vi "Dashboard Main.vi"() -> ()   [LabVIEW 2013]
uses:
  Vision/HSLRange.ctl
  <vilib>/event_ctls.llb/eventvkey.ctl
  <vilib>/Rock Robotics/WPI/Dashboard/WPI_DashboardLogging Global.vi
  <vilib>/Utility/config.llb/Write Key (String).vi
  <vilib>/Utility/config.llb/Write Key (I32).vi
  <vilib>/Utility/config.llb/NI_LVConfig.lvlib
panel:
  out "RobotIP":string
  out "Image Message":string="Timeout in Camera Communications"
  in  "Rec Mode":enum32{"Stop", "Record", "Playback"}(radio)
  in  "Dashboard Tab":T1(tab)
  in  "Camera Settings":T2={"Frame Rate"=30, "Compression"=30, "Size"=1} {"Frame Rate" scale=1.0..30.0; "Size" items=["640x480", "320x240", "160x120"]}
  out "MotorSliders R":cluster{"MotorSlide1":dbl, "MotorSlide2":dbl} {"MotorSlide2" scale=-1.0..1.0 scale format="%#_2e"; "MotorSlide1" scale=-1.0..1.0 scale format="%#_2e"}
  out "MotorChart R":cluster{"Numeric":dbl, "Numeric":dbl}(graph)
  out "MotorSliders L":T3 {"MotorSlide4 2" scale=0.0..14.0 scale format="%#_2e"; "MotorSlide2" scale=-1.0..1.0 scale format="%#_2e"; "MotorSlide1" scale=-1.0..1.0 scale format="%#_2e"}
  out "MotorChart L":T4(graph)
  out "JS1 Z":dbl(slide) scale=-1.0..1.0 scale format="%#_2e"
  out "Joystick 1":cluster{"X":dbl, "Y":dbl}[](graph)
  out "JS Buttons 1":T5
  out "JS2 Z":dbl(slide) scale=-1.0..1.0 scale format="%#_2e"
  out "Joystick 2":cluster{"X":dbl, "Y":dbl}[](graph)
  out "JS Buttons 2":T5
  out "Mode":T6(ring)=enum."Auto Disabled"
  out "Camera IP":string
  in  "DB Camera Config":bool
  out "fps":dbl format="%#.1g"
  out "Mbps":dbl format="%#.1g"
  out "Mbps 2":bool
  out "LED 1":bool
  in  "Score Limit":dbl
  in  "Minimum Area":dbl
  in  "HSL Range":T7={"Hue"={0.0, 130.10204081632654}, "Saturation"={111.88775510204081, 255.0}, "Luminance"={205.5612244897959, 255.0}} {"Luminance" scale=0.0..255.0; "Saturation" scale=0.0..255.0; "Hue" scale=0.0..255.0}
  in  "Checkbox 2":bool
  in  "Checkbox 1":bool
  in  "Test Slider":dbl(slide) scale=0.0..100.0 scale format="%#_3g"
  in  "On/Off":bool caption="Solenoid"
  in  "Test Name":u16(ring) items=["Select the test to run...", "Example Test", "-------------------------------", "List of tests is built in robot code.", "Replace with your own automated tests."]
  in  "Test Tree":string(tree)
  in  "Motor":cluster{"Value":dbl, "Enable":bool} {"Value" scale=-1.0..1.0 scale format="%#_3g"}
  out "Progress":T8 {"Test Progress" scale=0.0..100.0}
  in  "Rev/Fwd":cluster{"Forward":bool, "Reverse":bool}
  in  "Test Ring":u16(ring) items=["Auto", "Fixed indoor", "Fixed outdoor 1", "Fixed outdoor 2", "Fixed fluorescent 1", "Fixed fluorescent 2", "Hold current"]
  in  "Listbox":i32(listbox)
  out "Tree":string(tree)
  out "Camera Image":T9(plugin-control)
  in  "Enable":bool
  # "Left"
  # "Front"
  # "Right"
  # "Battery"
  # "Customize by placing controls and indicators here and name to\nmatch Dashboard Variables on robot."
  # "This tab is a great place for autonomous settings and validation.\nCustomize by placing controls and indicators here and name to\nmatch Dashboard Variables on robot."
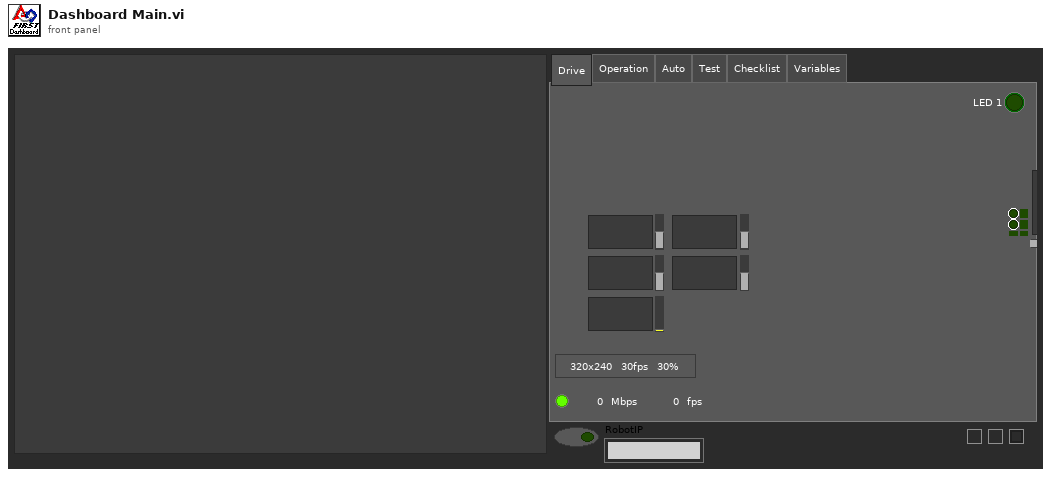
[diagram p1: front panel]
types:
  T1 = enum32{"Drive", "Operation", "Auto", "Test", "Checklist", "Variables"}
  T2 = cluster{"Frame Rate":i32, "Compression":i32, "Size":u16}
  T3 = cluster{"MotorSlide1":dbl, "MotorSlide2":dbl, "MotorSlide4 2":dbl}
  T4 = cluster{"Numeric":dbl, "Numeric":dbl, "Battery":sgl}
  T5 = cluster{bool, bool, bool, bool, bool, bool, bool, bool, bool, bool, bool, bool}
  T6 = enum8{"Tele-Op Disabled", "Tele-Op Enabled", "Auto Disabled", "Auto Enabled", "Test Disabled", "Test Enabled", ""}
  T7 = typedef "HSLRange.ctl" = cluster{"Hue":cluster{dbl, dbl}, "Saturation":cluster{dbl, dbl}, "Luminance":cluster{dbl, dbl}}
  T8 = cluster{"Test Progress":u8, "Test Progress Text":string}
  T9 = typedef "IMAQ Image.ctl" = refnum<image>
  T10 = typedef "Image Type" = u32
  T11 = typedef "Targetsss.ctl" = cluster{"Vertical Target":T12, "Horizontal Target":T12, "Valid?":bool, "Scores":T13, "Hot?":bool}
  T12 = typedef "Target Type.ctl" = cluster{"Area":dbl, "Bounding box":cluster{"BB Left":dbl, "BB Top":dbl, "BB Right":dbl, "BB Bottom":dbl}, "Center of Mass":cluster{"X Value":dbl, "Y Value":dbl}, "Equivilent Rectangle":cluster{"Width":dbl, "Height":dbl}, "Aspect Ratio":dbl, "Rectangularity":dbl, "Horizontal?":bool}
  T13 = typedef "Scores.ctl" = cluster{"Score Total":dbl, "Left Score":dbl, "Right Score":dbl, "Vertical Score":dbl, "Index":dbl}
  T14 = cluster{"BB Left":dbl, "BB Top":dbl, "BB Right":dbl, "BB Bottom":dbl}
  T15 = cluster{"Digital Inputs":bool[], "Digital Outputs":bool[]}
  T16 = cluster{"Competition mode":bool, "Robot Link":bool, "Autonomous":bool, "Enabled":bool, "E-Stop":bool, "Simulated":bool, "TestMode":bool, "Docked Window":bool}
  T17 = cluster{"Boolean Array[0]":bool, "Boolean Array[1]":bool, "Boolean Array[2]":bool, "Boolean Array[3]":bool, "Boolean Array[4]":bool, "Boolean Array[5]":bool, "Boolean Array[6]":bool, "Boolean Array[7]":bool, "Boolean Array[8]":bool, "Boolean Array[9]":bool, "Boolean Array[10]":bool, "Boolean Array[11]":bool}
  T18 = typedef "NI_LVConfig.lvlib/Config Data RefNum.ctl" = refnum<k1>
  T19 = typedef "eventvkey.ctl" = enum16{"ASCII", "Enter", "Return", "Shift", "Ctrl", "Alt", "Cmd", "Opt", "Caps", "NumLock", "Clear", "Break", "Up", "Down", "Left", "Right", "Insert", "Delete", "Home", "End", "PageUp", "PageDown", "Escape", "Help", "Pause", "ScrollLock", "F1", "F2", "F3", "F4", "F5", "F6", "F7", "F8", "F9", "F10", "F11", "F12", "F13", "F14", "F15", "F16", "F17", "F18", "F19", "F20", "F21", "F22", "F23", "F24", "Play", "VolumeUp", "VolumeDown", "Mute", "Two Byte Char"}
  T20 = cluster{"Image Size":bool, "Image Type":bool, "Pixel Value":bool, "ROI Information":bool, "Zoom Factor":bool}
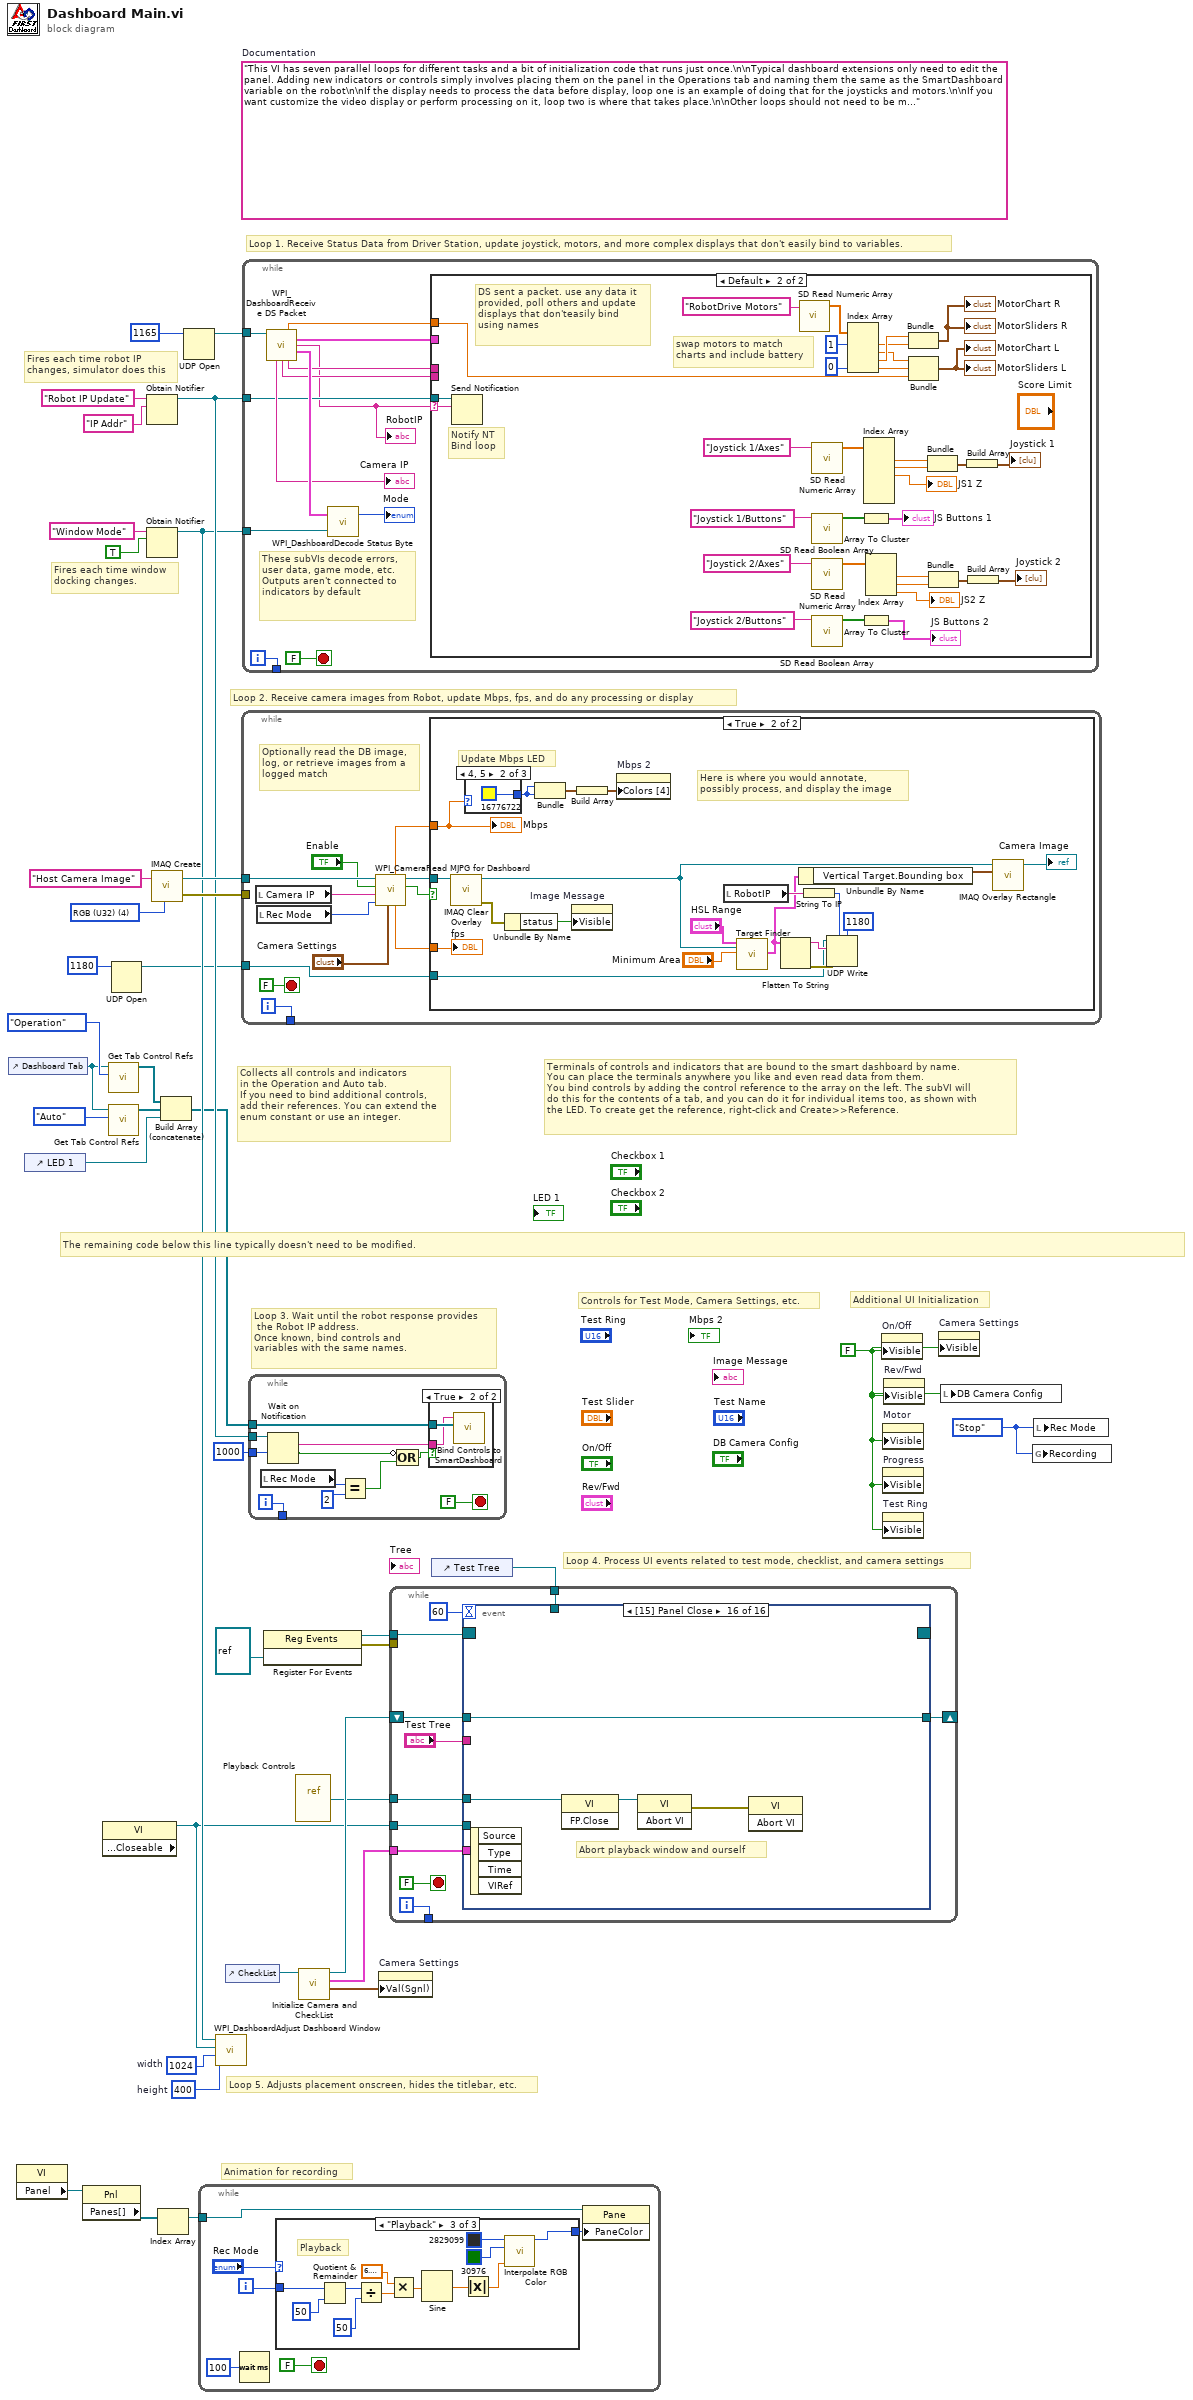
[diagram p0: block diagram]
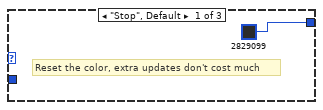
[diagram p2: hidden frame]
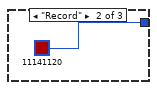
[diagram p3: hidden frame]
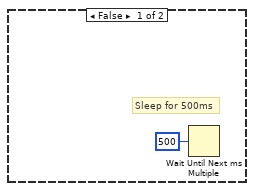
[diagram p5: hidden frame]
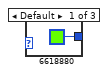
[diagram p6: hidden frame]
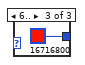
[diagram p7: hidden frame]
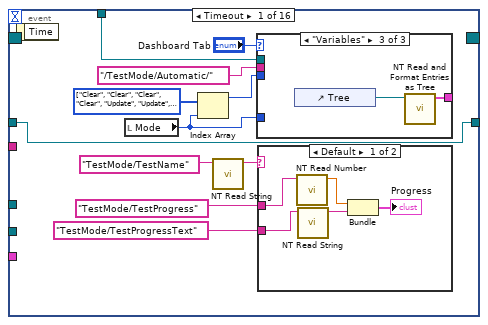
[diagram p8: hidden frame]
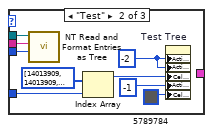
[diagram p10: hidden frame]
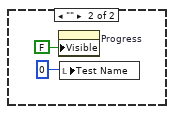
[diagram p11: hidden frame]
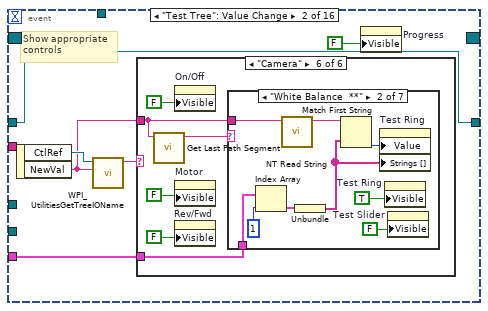
[diagram p12: hidden frame]
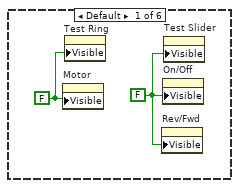
[diagram p13: hidden frame]
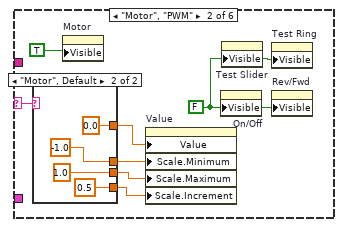
[diagram p14: hidden frame]
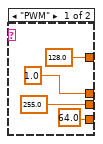
[diagram p15: hidden frame]
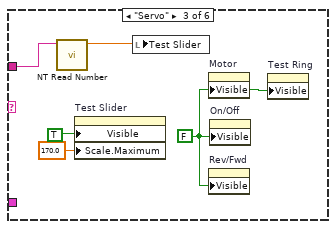
[diagram p16: hidden frame]
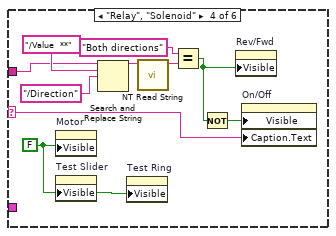
[diagram p17: hidden frame]
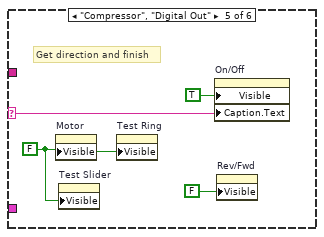
[diagram p18: hidden frame]
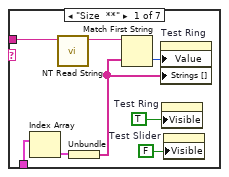
[diagram p19: hidden frame]
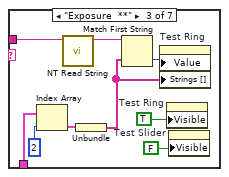
[diagram p20: hidden frame]
diagram:
  w10 = enum32{"Stop", "Record", "Playback"}."Stop" ("Rec Mode")
  w13 = 400  # height
  w14 = 1024  # width
  w27 = FALSE ("Visible")
  (unwired) "This VI has seven parallel loops for different tasks and a bit of initialization code that runs just once.\n\nTypical dashboard extensions only need to edit the panel. Adding new indicators or controls simply involves placing them on the panel in the Operations tab and naming them the same as the SmartDashboard variable on the robot\n\nIf the display needs to process the data before display, loop one is an example of doing that for the joysticks and motors.\n\nIf you want customize the video display or perform processing on it, loop two is where that takes place.\n\nOther loops should not need to be modified. They are pretty standard, and document the task they perform."  # Documentation
  w37 = T10 4 items=["Grayscale (U8)", "Grayscale (I16)", "Grayscale (SGL)", "Complex (CSG)", "RGB (U32)", "HSL (U32)", "RGB (U64)"] ("Image Type")
  # "Controls for Test Mode, Camera Settings, etc."
  # "Additional UI Initialization"
  # "Animation for recording"
  # "Fires each time robot IP\nchanges, simulator does this"
  # "Fires each time window\ndocking changes."
  # "Collects all controls and indicators\nin the Operation and Auto tab.\nIf you need to bind additional controls,\nadd their references. You can extend the\nenum constant or use an integer."
  # "The remaining code below this line typically doesn't need to be modified."
  # "Loop 4. Process UI events related to test mode, checklist, and camera settings"
  # "Terminals of controls and indicators that are bound to the smart dashboard by name.\nYou can place the terminals anywhere you like and even read data from them.\nYou bind controls by adding the control reference to the array on the left. The subVI will\ndo this for the contents of a tab, and you can do it for individual items too, as shown with\nthe LED. To create get the reference, right-click and Create>>Reference."
  # "Loop 3. Wait until the robot response provides\n the Robot IP address.\nOnce known, bind controls and\nvariables with the same names."
  # "Loop 5. Adjusts placement onscreen, hides the titlebar, etc."
  # "Loop 1. Receive Status Data from Driver Station, update joystick, motors, and more complex displays that don't easily bind to variables."
  # "Loop 2. Receive camera images from Robot, update Mbps, fps, and do any processing or display"
  n1 = control-ref of="Dashboard Tab"() -> (w8:refnum<vi>)
  n2 = property class="VI"() -> ("Panel"=w21:refnum<vi>)  [unwired: 2 in, 2 out]
  n3 = control-ref of="LED 1"() -> (w3:refnum<vi>)
  n4 = property class="Pnl"(reference=w21) -> ("Panes[]"=w22:refnum<vi>[])  [unwired: 1 in, 2 out]
  n5 = property class="VI" props=["Front Panel.Closeable"]() -> (reference out=w9:refnum<vi>)  [unwired: 2 in, 2 out]
  n6 = call <vilib>:"Get Tab Control Refs.vi"("Page Index"=T1."Operation" ("Dashboard Tab"), "TabControl in"=w8) -> ("ControlsOnPage"=w6:refnum<vi>[])  [unwired: 9 in]
  n7 = call <vilib>:"Get Tab Control Refs.vi"("Page Index"=T1."Auto" ("Dashboard Tab"), "TabControl in"=w8) -> ("ControlsOnPage"=w7:refnum<vi>[])  [unwired: 9 in]
  n8 = UDP Open(11:1180) -> (port=w2:refnum<k16>)  [unwired: 4 in, 2 out]
  n9 = Obtain Notifier(name (unnamed)="Robot IP Update", notification data type="IP Addr" ("name (unnamed)")) -> (notifier out=w31:refnum<notifier>)  [unwired: 2 in, 2 out]
  n10 = Obtain Notifier(name (unnamed)="Window Mode", notification data type=TRUE) -> (notifier out=w12:refnum<notifier>)  [unwired: 2 in, 2 out]
  n11 = call "IMAQ Create"("Image Name"="Host Camera Image", "Image Type"=w37) -> ("New Image"=w35:T9, "error out"=w34:errorcluster)  [unwired: 2 in, 1 out]
  n12 = Index Array(array=w22) -> (element=w20:refnum<vi>)  [unwired: 1 in]
  n13 = Build Array (concatenate)(w6, w7, w3) -> (w5:refnum<vi>[])
  n14 = UDP Open(11:u16 1165 ("port")) -> (port=w38:refnum<k16>)  [unwired: 2 in, 4 out]
  n15 = while {
    tunnel: w20 -> [w41]
    i -> [w44]
    stop <- FALSE stop-if-true
    n16 = Wait (ms)(milliseconds to wait=u32 100) -> ()  [unwired: 1 out]
    n17 = case shown="\"Playback\"" "Rec Mode" {
      tunnel: w44 -> [_ _ w59]
      tunnel: [u32 2829099 ("Base Color") u32 11141120 ("Target Color") w48] -> w40
      frame "Stop", Default {
        # "Reset the color, extra updates don't cost much"
      }
      frame "Record" {
      }
      frame "Playback" {
        # "Playback"
        n18 = Quotient & Remainder(x=w59, y=u32 50 ("milliseconds to wait")) -> (x-y*floor(x/y)=w55:u32)  [unwired: 1 out]
        n19 = Divide(x=w55, y=u32 50 ("milliseconds to wait")) -> (x/y=w52:dbl)
        n20 = Multiply(x=6.283185307179586, y=w52) -> (x*y=w57:dbl)
        n21 = Sine(x=w57) -> (sin(x)=w56:dbl)
        n22 = Absolute Value(x=w56) -> (abs(x)=w49:dbl)
        n23 = call "Interpolate RGB Color.vi"("Proportion"=w49, "Target Color"=u32 30976, "Base Color"=u32 2829099) -> ("Result Color"=w48:u32)  [unwired: 8 in]
      }
    }
    n24 = property class="Pane"(reference=w41, "PaneColor"=w40) -> ()  [unwired: 1 in, 2 out]
  }
  n25 = call <vilib>:"WPI_DashboardAdjust Dashboard Window.vi"("height"=w13, "width"=w14, "reference in"=w9, "Notifier in"=w12) -> ()  [unwired: 8 in]
  n26 = control-ref of="CheckList"() -> (w11:refnum<vi>)
  n27 = while {
    tunnel: w35 -> [w69]
    tunnel: w34 -> [_]
    tunnel: [w70] -> _
    tunnel: w2 -> [w60]
    i -> [w70]
    stop <- FALSE stop-if-true
    # "Optionally read the DB image,\nlog, or retrieve images from a\nlogged match"
    n28 = local read "Camera IP"() -> (w62:string)
    n29 = local read "Rec Mode"() -> (w61:enum32{"Stop", "Record", "Playback"})
    n30 = call <vilib>:"WPI_CameraRead MJPG for Dashboard.vi"("Camera Settings"="Camera Settings", "Rec Mode"=w61, "Camera IP"=w62, "Enable"="Enable", "Refnum in"=w69) -> ("Active"=w66:bool, "Refnum out"=w68:T9, "FPS"=w65:dbl, "Bandwidth (Mbps)"=w64:dbl)  [unwired: 3 in]
    n31 = case shown="True" w66 {
      tunnel: w68 -> [_ w87]
      tunnel: w64 -> [_ w86]
      tunnel: w65 -> [_ w85]
      tunnel: w60 -> [_ w81]
      frame False {
        # "Sleep for 500ms"
        n32 = Wait Until Next ms Multiple(millisecond multiple=u32 500) -> ()  [unwired: 1 out]
      }
      frame True {
        # "Here is where you would annotate,\npossibly process, and display the image"
        # "Update Mbps LED"
        n33 = call "IMAQ Clear Overlay"("Image"=w87) -> ("error out"=w91:errorcluster, "Image Out"=w77:T9)  [unwired: 2 in, 7 out]
        n34 = case shown="4, 5" w86 {
          tunnel: [u32 6618880 ("Color Box") u32 16776722 ("Color Box") u32 16716800 ("Color Box")] -> w88
          frame Default {
          }
          frame 4, 5 {
          }
          frame 6.. {
          }
        }
        n35 = Unbundle By Name(w91) -> ("status"=w92:bool)
        n36 = Bundle("Color Box"=w88, "Color Box"=w88) -> (w90:cluster{"Color Box":u32, "Color Box":u32})  [unwired: 1 out]
        n37 = property on="Image Message" class="Str"("Visible"=w92) -> ()  [unwired: 2 in, 2 out]
        n38 = Build Array(w90) -> (w89:cluster{"Color Box":u32, "Color Box":u32}[])
        n39 = property on="Mbps 2" class="Bool (strict)"("Colors [4]"=w89) -> ()  [unwired: 2 in, 2 out]
        n40 = local read "RobotIP"() -> (w78:string)
        n41 = call "Target Finder.vi"("HSL Range"="HSL Range", "Image"=w77, "Minimum Area"="Minimum Area") -> ("Targetssssss"=w74:T11)  [unwired: 16 in]
        n42 = Flatten To String(anything=w74) -> (data string=w82:string, error out=w83:errorcluster)  [unwired: 3 in, 1 out]
        n43 = Unbundle By Name(w74) -> ("Vertical Target.Bounding box"=w76:T14)
        n44 = String To IP(1:w78) -> (0:w79:u32)
        n45 = UDP Write(address=w79, port or service name=1180, connection ID=w81, data in=w82, 8:w83) -> ()  [unwired: 1 in, 2 out]
        n46 = call "IMAQ Overlay Rectangle"("Rectangle"=w76, "Image"=w77) -> ("Image Out"=→"Camera Image":T9)  [unwired: 8 in, 1 out]
        "Mbps" <- w86
        "fps" <- w85
      }
    }
  }
  n47 = while {
    tunnel: w38 -> [w106]
    tunnel: w31 -> [w101]
    tunnel: w12 -> [w105]
    tunnel: [w102] -> _
    i -> [w102]
    stop <- FALSE stop-if-true
    # "These subVIs decode errors, user data, game mode, etc.\nOutputs aren't connected to indicators by default"
    n48 = call <vilib>:"WPI_DashboardReceive DS Packet.vi"("Recv Socket"=w106) -> ("Battery"=w97:sgl, "Driver Station"=w98:T15, "Robot IP Address"=w96:string, "Status"=w107:T16, "Camera IP Address"=→"Camera IP":string, "Low Priority User Data"=w100:string, "High Priority User Data"=w99:string)  [unwired: 1 in, 7 out]
    "RobotIP" <- w96
    n49 = call <vilib>:"WPI_DashboardDecode Status Byte.vi"("Window Mode Notifier"=w105, "Status"=w107) -> ("Mode"=→"Mode":T6)  [unwired: 1 out]
    n50 = case shown="Default" w96 {
      selector: w96 -> [_ w119]
      tunnel: w101 -> [_ w120]
      tunnel: w100 -> [_ _]
      tunnel: w99 -> [_ _]
      tunnel: w98 -> [_ _]
      tunnel: w97 -> [_ w118]
      frame "0.0.0.0" {
        # "DS not sending packets, or no robot exists yet.\nDon't poll the variables"
      }
      frame Default {
        # "Notify NT\nBind loop"
        # "DS sent a packet. use any data it\nprovided, poll others and update\ndisplays that don'teasily bind\nusing names"
        # "swap motors to match\ncharts and include battery"
        n51 = Send Notification(notification=w119, notifier=w120) -> ()  [unwired: 1 in, 2 out]
        n52 = call <vilib>:"SD Read Numeric Array.vi"("Name"="RobotDrive Motors") -> ("Numeric Array"=w117:dbl[])  [unwired: 8 in, 2 out]
        n53 = call <vilib>:"SD Read Numeric Array.vi"("Name"="Joystick 1/Axes") -> ("Numeric Array"=w136:dbl[])  [unwired: 8 in, 2 out]
        n54 = call <vilib>:"SD Read Boolean Array.vi"("Name"="Joystick 1/Buttons") -> ("Boolean Array"=w138:bool[])  [unwired: 8 in, 2 out]
        n55 = call <vilib>:"SD Read Numeric Array.vi"("Name"="Joystick 2/Axes") -> ("Numeric Array"=w130:dbl[])  [unwired: 8 in, 2 out]
        n56 = call <vilib>:"SD Read Boolean Array.vi"("Name"="Joystick 2/Buttons") -> ("Boolean Array"=w129:bool[])  [unwired: 8 in, 2 out]
        n57 = Index Array(array=w117, index #1=1, index #4=0) -> (element #1=w113:dbl, element #2=w112:dbl, element #3=w114:dbl, element #4=w109:dbl)  [unwired: 2 in]
        n58 = Array To Cluster(array=w138) -> (cluster=→"JS Buttons 1":T17)
        n59 = Array To Cluster(array=w129) -> (cluster=→"JS Buttons 2":T17)
        n60 = Index Array(array=w136) -> (element #1=w133:dbl, element #2=w134:dbl, element #3=→"JS1 Z":dbl)  [unwired: 6 in, 3 out]
        n61 = Index Array(array=w130) -> (element #1=w125:dbl, element #2=w124:dbl, element #3=→"JS2 Z":dbl)  [unwired: 3 in]
        n62 = Bundle("Numeric"=w114, "Numeric"=w113) -> (→"MotorChart R" →"MotorSliders R":cluster{"Numeric":dbl, "Numeric":dbl})  [unwired: 1 in]
        n63 = Bundle("Numeric"=w112, "Numeric"=w109, "Battery"=w118) -> (→"MotorChart L" →"MotorSliders L":T4)  [unwired: 1 in]
        n64 = Bundle("Numeric"=w133, "Numeric"=w134) -> (w132:cluster{"Numeric":dbl, "Numeric":dbl})  [unwired: 1 in]
        n65 = Bundle("Numeric"=w125, "Numeric"=w124) -> (w126:cluster{"Numeric":dbl, "Numeric":dbl})  [unwired: 1 in]
        n66 = Build Array(w132) -> (→"Joystick 1":cluster{"Numeric":dbl, "Numeric":dbl}[])
        n67 = Build Array(w126) -> (→"Joystick 2":cluster{"Numeric":dbl, "Numeric":dbl}[])
      }
    }
  }
  n68 = while {
    tunnel: w5 -> [w152]
    tunnel: w31 -> [w150]
    tunnel: [w148] -> _
    tunnel: u32 1000 ("milliseconds to wait") -> [w147]
    i -> [w148]
    stop <- FALSE stop-if-true
    n69 = local read "Rec Mode"() -> (w143:enum32{"Stop", "Record", "Playback"})
    n70 = Wait on Notification(notifier=w150, timeout in ms (-1)=w147) -> (notification=w149:string, timed out?=w145:bool)  [unwired: 2 in, 2 out]
    n71 = Equal?(x=w143, y=u16 2 ("Rec Mode")) -> (x = y?=w144:bool)
    n72 = Compound Arithmetic op=OR(invert w145, w144) -> (w146:bool)
    n73 = case shown="True" w146 {
      tunnel: w152 -> [_ w154]
      tunnel: w149 -> [_ w153]
      frame False {
      }
      frame True {
        n74 = call <vilib>:"Bind Controls to SmartDashboard.vi"("Bound Control Refs"=w154, "Server IP Address"=w153) -> ()  [unwired: 10 in]
      }
    }
  }
  n75 = register-events(refnum<vi> refnum) -> (reference out=w18:refnum<event-registration>, error out=w17:errorcluster)  [unwired: 2 in]
  n76 = vi-ref "Playback Controls.vi"() -> (w19:refnum<vi>)
  n77 = call "Initialize Camera and CheckList.vi"("ListBox in"=w11) -> ("Cluster"=w25:cluster{"value":i32, "value":i32, "index":i32}, "Array"=w26:cluster{string[]}[], "File Refnum"=w24:T18)  [unwired: 8 in]
  n78 = property on="Camera Settings" class="Clust (strict)"("Val(Sgnl)"=w25) -> ()  [unwired: 2 in, 2 out]
  n79 = control-ref of="Test Tree"() -> (w23:refnum<vi>)
  n80 = while {
    tunnel: w26 -> [w162]
    shift-right: [w161] -> _
    shift-left: w24 -> [w160]
    tunnel: [w159] -> _
    tunnel: w23 -> [w158]
    tunnel: w19 -> [w157]
    tunnel: w18 -> [w156]
    tunnel: w17 -> [_]
    tunnel: w9 -> [w155]
    i -> [w159]
    stop <- FALSE stop-if-true
    n81 = event shown="[15] Panel Close" {
      selector: w156 -> [_ _ _ _ _ _ _ _ _ _ _ _ _ _ _ _]
      dyn-events: [_ _ _ _ _ _ _ _ _ _ _ _ _ w400 _ _] -> _
      timeout: u32 60 ("milliseconds to wait") -> [_ _ _ _ _ _ _ _ _ _ _ _ _ _ _ _]
      tunnel: w158 -> [w172 _ _ _ _ _ _ _ _ _ _ _ _ _ _ _]
      tunnel: "Test Tree" -> [_ _ _ _ _ _ _ _ w369 w377 w379 w383 w391 _ _ _]
      tunnel: w162 -> [_ w196 _ _ _ _ w333 w363 _ _ _ _ _ _ _ _]
      tunnel: [w166 w195 w294 w299 w307 w319 w332 w356 w368 w375 w378 w382 w390 w402 w416 w417] -> w161
      tunnel: w160 -> [w166 w195 w294 w299 w307 w319 w331 w356 w368 w375 w378 w382 w390 w402 w416 w417]
      tunnel: w157 -> [_ _ _ _ _ _ _ _ _ _ _ _ _ w403 _ w420]
      tunnel: w155 -> [_ _ _ _ _ _ _ _ _ _ _ _ _ w398 _ _]
      event Timeout {
        w171 = enum16{"Update", "Clear"}[] [enum."Clear", enum."Clear", enum."Clear", enum."Clear", enum."Update", enum."Update", enum."Clear"] items=["Update", "Clear"]
        n82 = event-data() -> ()  [unwired: 1 in, 1 out]
        n83 = local read "Mode"() -> (w169:T6)
        n84 = Index Array(array=w171, index=w169) -> (element=w170:enum16{"Update", "Clear"})
        n85 = call <vilib>:"NT Read String.vi"("Name"="TestMode/TestName") -> ("String"=w175:string)  [unwired: 9 in, 1 out]
        n86 = case shown="\"Variables\"" "Dashboard Tab" {
          tunnel: w172 -> [_ w185 _]
          tunnel: "/TestMode/Automatic/" ("Name Pattern") -> [_ w184 _]
          tunnel: w170 -> [_ w183 _]
          tunnel: w169 -> [_ w181 _]
          tunnel: [_ _ w187] -> _
          frame "Operation", Default {
          }
          frame "Test" {
            w180 = -2 ("Active Item:Row Number")
            n87 = call <vilib>:"NT Read and Format Entries as Tree.vi"("Operation"=w183, "Name Pattern"=w184, "Tree Refnum"=w185) -> ()  [unwired: 7 in, 2 out]
            n88 = Index Array(array=u32[] [14013909, 14013909, 14013909, 14013909, 14013909, 16777215, 14013909], index=w181) -> (element=w179:u32)
            n89 = property on="Test Tree" class="Tree (strict)"("Active Item Row Number"=w180, "ActiveColNum"=w180, "CellBG"=w179, "Active Item Row Number"=-1 ("Active Item:Row Number"), "CellBG"=u32 5789784 ("Color Box")) -> ()  [unwired: 2 in, 2 out]
          }
          frame "Variables" {
            n90 = control-ref of="Tree"() -> (w186:refnum<vi>)
            n91 = call <vilib>:"NT Read and Format Entries as Tree.vi"("Tree Refnum"=w186) -> ("Formatted Strings"=w187:cluster{"Name":string, "Value":string}[])  [unwired: 9 in, 1 out]
          }
        }
        n92 = case shown="Default" w175 {
          tunnel: "TestMode/TestProgress" ("Name") -> [w189 _]
          tunnel: "TestMode/TestProgressText" ("Name") -> [w188 _]
          frame Default {
            n93 = call <vilib>:"NT Read Number.vi"("Name"=w189) -> ("Numeric"=w190:dbl)  [unwired: 9 in, 1 out]
            n94 = call <vilib>:"NT Read String.vi"("Name"=w188) -> ("String"=w191:string)  [unwired: 9 in, 1 out]
            n95 = Bundle("Numeric"=w190, "String"=w191) -> (→"Progress":cluster{"Numeric":dbl, "String":string})  [unwired: 1 in]
          }
          frame "" {
            n96 = property on="Progress" class="Clust (strict)"("Visible"=FALSE) -> ()  [unwired: 2 in, 2 out]
            n97 = local write "Test Name"(u16 0) -> ()
          }
        }
      }
      event "Test Tree": Value Change {
        # "Show appropriate\ncontrols"
        n98 = event-data() -> ("CtlRef"=w199:refnum<vi>, "NewVal"=w197:string)  [unwired: 1 in]
        n99 = call <vilib>:"WPI_UtilitiesGetTreeIOName.vi"("NewVal"=w197, "TreeControl in"=w199) -> ("I/O Name"=w200:string)  [unwired: 9 in]
        n100 = case shown="\"Camera\"" w200 {
          selector: w200 -> [_ w207 _ w225 w234 _]
          tunnel: w197 -> [_ _ w222 w224 _ w241]
          tunnel: w196 -> [_ _ _ _ _ w240]
          frame Default {
            w202 = FALSE ("Visible")
            w201 = FALSE ("Visible")
            n101 = property on="Motor" class="Clust (strict)"("Visible"=w201) -> ()  [unwired: 2 in, 2 out]
            n102 = property on="Test Ring" class="Ring (strict)"("Visible"=w201) -> ()  [unwired: 2 in, 2 out]
            n103 = property on="Rev/Fwd" class="Clust (strict)"("Visible"=w202) -> ()  [unwired: 2 in, 2 out]
            n104 = property on="On/Off" class="Bool (strict)"("Visible"=w202) -> ()  [unwired: 2 in, 2 out]
            n105 = property on="Test Slider" class="Slide (strict)"("Visible"=w202) -> ()  [unwired: 2 in, 2 out]
          }
          frame "Motor", "PWM" {
            w208 = FALSE ("Visible")
            n106 = case shown="\"Motor\", Default" w207 {
              tunnel: [1.0 ("Value") -1.0 ("Value")] -> w206
              tunnel: [255.0 ("Value") 1.0 ("Value")] -> w205
              tunnel: [128.0 ("Value") 0.0 ("Value")] -> w204
              tunnel: [64.0 ("Value") 0.5 ("Value")] -> w203
              frame "PWM" {
              }
              frame "Motor", Default {
              }
            }
            n107 = property on="Motor" class="Clust (strict)"("Visible"=TRUE) -> ()  [unwired: 2 in, 2 out]
            n108 = property on="Value" class="Slide (strict)"("Value"=w204, "Scale.Minimum"=w206, "Scale.Maximum"=w205, "Scale.Increment"=w203) -> ()  [unwired: 2 in, 2 out]
            n109 = property on="On/Off" class="Bool (strict)"("Visible"=w208) -> ()  [unwired: 2 in, 2 out]
            n110 = property on="Test Slider" class="Slide (strict)"("Visible"=w208) -> ()  [unwired: 2 in, 2 out]
            n111 = property on="Test Ring" class="Ring (strict)"("Visible"=w208) -> ()  [unwired: 2 in, 2 out]
            n112 = property on="Rev/Fwd" class="Clust (strict)"("Visible"=w208) -> ()  [unwired: 2 in, 2 out]
          }
          frame "Servo" {
            w220 = FALSE ("Visible")
            n113 = call <vilib>:"NT Read Number.vi"("Name"=w222) -> ("Numeric"=w221:dbl)  [unwired: 9 in, 1 out]
            n114 = property on="Test Slider" class="Slide (strict)"("Visible"=TRUE, "Scale.Maximum"=170.0 ("Scale.Range:Maximum")) -> ()  [unwired: 2 in, 2 out]
            n115 = local write "Test Slider"(w221) -> ()
            n116 = property on="Motor" class="Clust (strict)"("Visible"=w220) -> ()  [unwired: 2 in, 2 out]
            n117 = property on="Rev/Fwd" class="Clust (strict)"("Visible"=w220) -> ()  [unwired: 2 in, 2 out]
            n118 = property on="On/Off" class="Bool (strict)"("Visible"=w220) -> ()  [unwired: 2 in, 2 out]
            n119 = property on="Test Ring" class="Ring (strict)"("Visible"=w220) -> ()  [unwired: 2 in, 2 out]
          }
          frame "Relay", "Solenoid" {
            w223 = FALSE ("Visible")
            n120 = property on="Motor" class="Clust (strict)"("Visible"=w223) -> ()  [unwired: 2 in, 2 out]
            n121 = property on="Test Slider" class="Slide (strict)"("Visible"=w223) -> ()  [unwired: 2 in, 2 out]
            n122 = Search and Replace String(input string=w224, search string="/Value  **", replace string="/Direction") -> (result string=w230:string)  [unwired: 5 in, 3 out]
            n123 = property on="Test Ring" class="Ring (strict)"("Visible"=w223) -> ()  [unwired: 2 in, 2 out]
            n124 = call <vilib>:"NT Read String.vi"("Name"=w230) -> ("String"=w228:string)  [unwired: 9 in, 1 out]
            n125 = Equal?(x="Both directions", y=w228) -> (x = y?=w226:bool)
            n126 = Not(x=w226) -> (.not. x?=w227:bool)
            n127 = property on="Rev/Fwd" class="Clust (strict)"("Visible"=w226) -> ()  [unwired: 2 in, 2 out]
            n128 = property on="On/Off" class="Bool (strict)"("Visible"=w227, "Caption.Text"=w225) -> ()  [unwired: 2 in, 2 out]
          }
          frame "Compressor", "Digital Out" {
            w233 = FALSE ("Visible")
            # "Get direction and finish"
            n129 = property on="Motor" class="Clust (strict)"("Visible"=w233) -> ()  [unwired: 2 in, 2 out]
            n130 = property on="Test Slider" class="Slide (strict)"("Visible"=w233) -> ()  [unwired: 2 in, 2 out]
            n131 = property on="Test Ring" class="Ring (strict)"("Visible"=w233) -> ()  [unwired: 2 in, 2 out]
            n132 = property on="On/Off" class="Bool (strict)"("Visible"=TRUE, "Caption.Text"=w234) -> ()  [unwired: 2 in, 2 out]
            n133 = property on="Rev/Fwd" class="Clust (strict)"("Visible"=FALSE) -> ()  [unwired: 2 in, 2 out]
          }
          frame "Camera" {
            n134 = call <vilib>:"Get Last Path Segment.vi"("String in"=w241) -> ("String out"=w242:string)  [unwired: 10 in]
            n135 = property on="On/Off" class="Bool (strict)"("Visible"=FALSE) -> ()  [unwired: 2 in, 2 out]
            n136 = property on="Motor" class="Clust (strict)"("Visible"=FALSE) -> ()  [unwired: 2 in, 2 out]
            n137 = property on="Rev/Fwd" class="Clust (strict)"("Visible"=FALSE) -> ()  [unwired: 2 in, 2 out]
            n138 = case shown="\"White Balance  **\"" w242 {
              tunnel: w241 -> [w248 w257 w266 w275 w284 _ w290]
              tunnel: w240 -> [w246 w254 w263 w272 w281 _ _]
              frame "Size  **" {
                n139 = Index Array(array=w246) -> (element=w245:cluster{string[]})  [unwired: 1 in]
                n140 = call <vilib>:"NT Read String.vi"("Name"=w248) -> ("String"=w247:string)  [unwired: 9 in, 1 out]
                n141 = Unbundle(w245) -> (w243:string[])
                n142 = Match First String(2:w243, 3:w247) -> (0:w244:i32)  [unwired: 1 out]
                n143 = property on="Test Ring" class="Ring (strict)"("Value"=w244, "Strings []"=w243) -> ()  [unwired: 2 in, 2 out]
                n144 = property on="Test Ring" class="Ring (strict)"("Visible"=TRUE) -> ()  [unwired: 2 in, 2 out]
                n145 = property on="Test Slider" class="Slide (strict)"("Visible"=FALSE) -> ()  [unwired: 2 in, 2 out]
              }
              frame "White Balance  **" {
                n146 = Index Array(array=w254, index=1) -> (element=w255:cluster{string[]})
                n147 = call <vilib>:"NT Read String.vi"("Name"=w257) -> ("String"=w256:string)  [unwired: 9 in, 1 out]
                n148 = Unbundle(w255) -> (w252:string[])
                n149 = Match First String(2:w252, 3:w256) -> (0:w251:i32)  [unwired: 1 out]
                n150 = property on="Test Ring" class="Ring (strict)"("Value"=w251, "Strings []"=w252) -> ()  [unwired: 2 in, 2 out]
                n151 = property on="Test Ring" class="Ring (strict)"("Visible"=TRUE) -> ()  [unwired: 2 in, 2 out]
                n152 = property on="Test Slider" class="Slide (strict)"("Visible"=FALSE) -> ()  [unwired: 2 in, 2 out]
              }
              frame "Exposure  **" {
                n153 = Index Array(array=w263, index=2) -> (element=w264:cluster{string[]})
                n154 = call <vilib>:"NT Read String.vi"("Name"=w266) -> ("String"=w265:string)  [unwired: 9 in, 1 out]
                n155 = Unbundle(w264) -> (w260:string[])
                n156 = Match First String(2:w260, 3:w265) -> (0:w261:i32)  [unwired: 1 out]
                n157 = property on="Test Ring" class="Ring (strict)"("Value"=w261, "Strings []"=w260) -> ()  [unwired: 2 in, 2 out]
                n158 = property on="Test Ring" class="Ring (strict)"("Visible"=TRUE) -> ()  [unwired: 2 in, 2 out]
                n159 = property on="Test Slider" class="Slide (strict)"("Visible"=FALSE) -> ()  [unwired: 2 in, 2 out]
              }
              frame "Exposure Priority  **" {
                n160 = Index Array(array=w272, index=3) -> (element=w273:cluster{string[]})
                n161 = call <vilib>:"NT Read String.vi"("Name"=w275) -> ("String"=w274:string)  [unwired: 9 in, 1 out]
                n162 = Unbundle(w273) -> (w269:string[])
                n163 = Match First String(2:w269, 3:w274) -> (0:w270:i32)  [unwired: 1 out]
                n164 = property on="Test Ring" class="Ring (strict)"("Value"=w270, "Strings []"=w269) -> ()  [unwired: 2 in, 2 out]
                n165 = property on="Test Ring" class="Ring (strict)"("Visible"=TRUE) -> ()  [unwired: 2 in, 2 out]
                n166 = property on="Test Slider" class="Slide (strict)"("Visible"=FALSE) -> ()  [unwired: 2 in, 2 out]
              }
              frame "Color Enable  **" {
                n167 = Index Array(array=w281, index=4) -> (element=w282:cluster{string[]})
                n168 = call <vilib>:"NT Read String.vi"("Name"=w284) -> ("String"=w283:string)  [unwired: 9 in, 1 out]
                n169 = Unbundle(w282) -> (w278:string[])
                n170 = Match First String(2:w278, 3:w283) -> (0:w279:i32)  [unwired: 1 out]
                n171 = property on="Test Ring" class="Ring (strict)"("Value"=w279, "Strings []"=w278) -> ()  [unwired: 2 in, 2 out]
                n172 = property on="Test Ring" class="Ring (strict)"("Visible"=TRUE) -> ()  [unwired: 2 in, 2 out]
                n173 = property on="Test Slider" class="Slide (strict)"("Visible"=FALSE) -> ()  [unwired: 2 in, 2 out]
              }
              frame Default {
                n174 = property on="Test Ring" class="Ring (strict)"("Visible"=FALSE) -> ()  [unwired: 2 in, 2 out]
                n175 = property on="Test Slider" class="Slide (strict)"("Visible"=FALSE) -> ()  [unwired: 2 in, 2 out]
              }
              frame "Brightness  **", "Color Level  **", "Compression  **", "FPS  **", "Sharpness  **" {
                n176 = call <vilib>:"NT Read Number.vi"("Name"=w290) -> ("Numeric"=w289:dbl)  [unwired: 9 in, 1 out]
                n177 = local write "Test Slider"(w289) -> ()
                n178 = property on="Test Slider" class="Slide (strict)"("Visible"=TRUE, "Scale.Maximum"=100.0 ("Scale.Range:Maximum")) -> ()  [unwired: 2 in, 2 out]
                n179 = property on="Test Ring" class="Ring (strict)"("Visible"=FALSE) -> ()  [unwired: 2 in, 2 out]
              }
            }
          }
        }
        n180 = property on="Progress" class="Clust (strict)"("Visible"=FALSE) -> ()  [unwired: 2 in, 2 out]
      }
      event "Test Name": Mouse Enter {
        # "Populate the ring with the list of tests"
        n181 = event-data() -> ()  [unwired: 1 in, 1 out]
        n182 = call <vilib>:"NT Read String Array.vi"("Name"="TestMode/TestList") -> ("String Array"=w298:string[])  [unwired: 9 in, 1 out]
        n183 = Build Array (concatenate)("Select the test to run...", w298) -> (w297:string[])
        n184 = property on="Test Name" class="Ring (strict)"("Strings []"=w297) -> ()  [unwired: 2 in, 2 out]
      }
      event "Test Name": Value Change {
        w300 = FALSE ("Visible")
        # "Tell the robot the test name to run"
        n185 = event-data() -> ("NewVal"=w304:u16)  [unwired: 1 in]
        n186 = property on="Test Name" class="Ring (strict)"() -> ("Strings []"=w305:string[])  [unwired: 2 in, 2 out]
        n187 = local write "Progress"(T8 {"Test Progress"=0, "Test Progress Text"=""} ("Progress")) -> ()
        n188 = Index Array(array=w305, index=w304) -> (element=w303:string)
        n189 = call <vilib>:"NT Write String.vi"("String"=w303, "Name"="TestMode/TestName") -> ()  [unwired: 9 in, 1 out]
        n190 = property on="Progress" class="Clust (strict)"("Visible"=TRUE) -> ()  [unwired: 2 in, 2 out]
        n191 = property on="Motor" class="Clust (strict)"("Visible"=w300) -> ()  [unwired: 2 in, 2 out]
        n192 = property on="Test Slider" class="Slide (strict)"("Visible"=w300) -> ()  [unwired: 2 in, 2 out]
        n193 = property on="On/Off" class="Bool (strict)"("Visible"=w300) -> ()  [unwired: 2 in, 2 out]
        n194 = property on="Rev/Fwd" class="Clust (strict)"("Visible"=w300) -> ()  [unwired: 2 in, 2 out]
        n195 = property on="Test Ring" class="Ring (strict)"("Visible"=w300) -> ()  [unwired: 2 in, 2 out]
      }
      event "Listbox": Double Click {
        n196 = event-data() -> ("PlatMods.Shift"=w308:bool, "Row"=w310:i32)  [unwired: 1 in]
        n197 = case shown="True" w308 {
          tunnel: w310 -> [w314 _]
          tunnel: 1 -> [w313 _]
          frame False {
            n198 = property on="Listbox" class="LstBox (strict)"() -> ("Item Symbols"=w312:i32[])  [unwired: 2 in, 2 out]
            n199 = Replace Array Subset(array=w312, new element=w313, index=w314) -> (w311:i32[])
            n200 = property on="Listbox" class="LstBox (strict)"("Item Symbols"=w311) -> ()  [unwired: 2 in, 2 out]
          }
          frame True {
            w315 = 0 ("Top Row")
            n201 = property on="Listbox" class="LstBox (strict)"() -> ("Number of Rows"=w317:u32)  [unwired: 2 in, 2 out]
            n202 = Initialize Array(0, w317) -> (w316:i32[])
            n203 = property on="Listbox" class="LstBox (strict)"("Top Row"=w315, "Value"=w315, "Item Symbols"=w316) -> ()  [unwired: 2 in, 2 out]
          }
        }
      }
      event "Listbox": Key Down {
        n204 = event-data() -> ("VKey"=w321:T19)  [unwired: 1 in]
        n205 = case shown="\"Left\", \"Right\"" w321 {
          selector: w321 -> [w326 _]
          tunnel: eventvkey."Left" ("VKey") -> [w324 _]
          frame "Left", "Right" {
            n206 = Equal?(x=w324, y=w326) -> (x = y?=w325:bool)
            n207 = Select(t=0, s=w325, f=1) -> (s? t:f=w327:i32)
            n208 = property on="Listbox" class="LstBox (strict)"() -> ("Item Symbols"=w330:i32[])  [unwired: 2 in, 2 out]
            n209 = Replace Array Subset(array=w330, new element=w327, index="Listbox") -> (w329:i32[])
            n210 = property on="Listbox" class="LstBox (strict)"("Item Symbols"=w329) -> ()  [unwired: 2 in, 2 out]
          }
          frame Default {
          }
        }
      }
      event "DB Camera Config": Value Change {
        n211 = event-data() -> ("NewVal"=w334:bool)  [unwired: 1 in]
        n212 = case shown="False" w334 {
          tunnel: w333 -> [w343 _]
          tunnel: [w336 w354] -> w332
          tunnel: w331 -> [w335 w354]
          frame False {
            w350 = "Camera"
            w353 = FALSE ("Visible")
            n213 = local read "Camera Settings"() -> (w342:T2)
            n214 = Index Array(array=w343) -> (element=w346:cluster{string[]})  [unwired: 1 in]
            n215 = Unbundle(w342) -> ("Frame Rate"=w341:i32, "Compression"=w340:i32, "Size"=w344:u16)
            n216 = Unbundle(w346) -> (w345:string[])
            n217 = Index Array(array=w345, index=w344) -> (element=w339:string)
            n218 = call-poly <vilib>:"Write Key.vi"("section"=w350, "value"=w339, "key"="Size", "refnum"=w335) -> ("refnum out"=w352:T18)  [unwired: 2 in, 5 out]
            n219 = call-poly <vilib>:"Write Key.vi"("section"=w350, "value"=w341, "key"="FrameRate", "refnum"=w352) -> ("refnum out"=w351:T18)  [unwired: 1 in, 6 out]
            n220 = property on="Camera Settings" class="Clust (strict)"("Visible"=w353) -> ()  [unwired: 2 in, 2 out]
            n221 = local write "DB Camera Config"(w353) -> ()
            n222 = call-poly <vilib>:"Write Key.vi"("section"=w350, "value"=w340, "key"="Compression", "refnum"=w351) -> ("refnum out"=w337:T18)  [unwired: 1 in, 6 out]
            n223 = call <vilib>:"Close Config Data.vi"("refnum"=w337) -> ("file path"=w338:path)  [unwired: 2 in, 8 out]
            n224 = call <vilib>:"Open Config Data.vi"("configuration file path"=w338) -> ("refnum"=w336:T18)  [unwired: 8 in, 2 out]
          }
          frame True {
            n225 = property on="Camera Settings" class="Clust (strict)"("Visible"=TRUE) -> ()  [unwired: 2 in, 2 out]
          }
        }
      }
      event "Camera Settings": Value Change {
        n226 = event-data() -> ("NewVal"=w367:T2)  [unwired: 1 in]
        n227 = Index Array(array=w363) -> (element=w362:cluster{string[]})  [unwired: 1 in]
        n228 = Unbundle(w367) -> ("Frame Rate"=w358:i32, "Compression"=w357:i32, "Size"=w360:u16)
        n229 = Unbundle(w362) -> (w361:string[])
        n230 = Index Array(array=w361, index=w360) -> (element=w359:string)
        n231 = Format Into String(format string="%s   %dfps   %d%%", w359, w358, w357) -> (resulting string=w364:string)  [unwired: 2 in, 1 out]
        n232 = Build Array(w364) -> (w365:string[])
        n233 = property on="DB Camera Config" class="Bool (strict)"("Strings [4]"=w365) -> ()  [unwired: 2 in, 2 out]
      }
      event "Motor.Enable": Value Change {
        n234 = event-data() -> ("NewVal"=w373:bool)  [unwired: 1 in]
        n235 = Unbundle("Motor") -> ("Value"=w372:dbl)  [unwired: 1 out]
        n236 = Select(t=w372, s=w373, f=0.0) -> (s? t:f=w370:dbl)
        n237 = call <vilib>:"NT Write Number.vi"("Numeric"=w370, "Name"=w369) -> ()  [unwired: 9 in, 1 out]
      }
      event "Test Slider": Value Change {
        n238 = event-data() -> ("NewVal"=w376:dbl)  [unwired: 1 in]
        n239 = call <vilib>:"NT Write Number.vi"("Numeric"=w376, "Name"=w377) -> ()  [unwired: 9 in, 1 out]
      }
      event "On/Off": Value Change {
        n240 = event-data() -> ("NewVal"=w381:bool)  [unwired: 1 in]
        n241 = Boolean To (0,1)(Boolean=w381) -> (0, 1=w380:i16)
        n242 = call <vilib>:"NT Write Number.vi"("Numeric"=w380, "Name"=w379) -> ()  [unwired: 9 in, 1 out]
      }
      event "Rev/Fwd": Value Change {
        n243 = event-data() -> ("NewVal.Forward"=w389:bool, "NewVal.Reverse"=w388:bool)  [unwired: 1 in]
        n244 = Boolean To (0,1)(Boolean=w389) -> (0, 1=w385:i16)
        n245 = Boolean To (0,1)(Boolean=w388) -> (0, 1=w387:i16)
        n246 = Negate(x=w387) -> (-x=w386:i16)
        n247 = Add(x=w385, y=w386) -> (x+y=w384:i16)
        n248 = call <vilib>:"NT Write Number.vi"("Numeric"=w384, "Name"=w383) -> ()  [unwired: 9 in, 1 out]
      }
      event "Test Ring": Value Change {
        n249 = event-data() -> ("NewVal"=w393:u16)  [unwired: 1 in]
        n250 = property on="Test Ring" class="Ring (strict)"() -> ("Strings []"=w394:string[])  [unwired: 2 in, 2 out]
        n251 = Index Array(array=w394, index=w393) -> (element=w392:string)
        n252 = call <vilib>:"NT Write String.vi"("String"=w392, "Name"=w391) -> ()  [unwired: 9 in, 1 out]
      }
      event "Rec Mode": Value Change {
        # "Update globals for recording mode and path to read log from.\nClear when logging and let NetworkTables set path for vision to\nuse."
        n253 = event-data() -> ("NewVal"=w404:enum32{"Stop", "Record", "Playback"})  [unwired: 1 in]
        n254 = global write "WPI_DashboardLogging Global.vi" "Logging Filename"(path "") -> ()
        n255 = case shown="\"Stop\", \"Record\"" w404 {
          tunnel: w403 -> [_ w406 w414]
          tunnel: [_ _ w413] -> w400
          tunnel: [_ _ w412] -> _
          tunnel: w398 -> [_ _ w410]
          tunnel: cluster{i32, i32} {-250, 170} -> [_ _ w409]
          tunnel: [_ _ T20 {"Image Size"=TRUE, "Image Type"=TRUE, "Pixel Value"=TRUE, "ROI Information"=TRUE, "Zoom Factor"=FALSE} ("Image Information Shown:All Elements")] -> w396
          tunnel: [_ _ TRUE ("Zoom Factor")] -> w395
          frame Default {
          }
          frame "Stop", "Record" {
            # "Place Window too"
            n256 = invoke class="VI" method="FP.Close"(reference=w406) -> (reference out=w405:refnum<vi>)  [unwired: 2 in, 2 out]
            n257 = invoke class="VI" method="Abort VI"(reference=w405) -> ()  [unwired: 2 in, 3 out]
          }
          frame "Playback" {
            n258 = call "Open Playback Panel.vi"("Offset"=w409, "DB VI Ref"=w410, "Playback in"=w414) -> ("Playback out"=w411:refnum<vi>)  [unwired: 8 in]
            n259 = register-events(w411) -> (reference out=w413:refnum<event-registration>, error out=w412:errorcluster)  [unwired: 2 in]
          }
        }
        n260 = global write "WPI_DashboardLogging Global.vi" "Recording"(w404) -> ()
        n261 = property on="Camera Image" class="ImageControl"("Image Information Shown"=w396, "Image Information Visible"=w395) -> ()  [unwired: 2 in, 2 out]
        n262 = call <vilib>:"WPI_DashboardNT Log FieldName Cache.vi"("Operation"=enum16{"Lookup/Add", "Index", "Clear"}."Clear") -> ()  [unwired: 8 in, 3 out]
      }
      event Panel Close {
        w415 = enum32{"Stop", "Record", "Playback"}."Stop" ("Rec Mode")
        n263 = event-data() -> ()  [unwired: 1 in, 4 out]
        n264 = local write "Rec Mode"(w415) -> ()
        n265 = global write "WPI_DashboardLogging Global.vi" "Recording"(w415) -> ()
      }
      event Panel Close {
        # "Abort playback window and ourself"
        n266 = event-data() -> ()  [unwired: 1 in, 4 out]
        n267 = invoke class="VI" method="FP.Close"(reference=w420) -> (reference out=w419:refnum<vi>)  [unwired: 2 in, 2 out]
        n268 = invoke class="VI" method="Abort VI"(reference=w419) -> (error out=w418:errorcluster)  [unwired: 2 in, 2 out]
        n269 = invoke class="VI" method="Abort VI"(error in=w418) -> ()  [unwired: 2 in, 3 out]
      }
    }
  }
  n270 = property on="On/Off" class="Bool (strict)"("Visible"=w27) -> ()  [unwired: 2 in, 2 out]
  n271 = property on="Motor" class="Clust (strict)"("Visible"=w27) -> ()  [unwired: 2 in, 2 out]
  n272 = property on="Progress" class="Clust (strict)"("Visible"=w27) -> ()  [unwired: 2 in, 2 out]
  n273 = property on="Test Ring" class="Ring (strict)"("Visible"=w27) -> ()  [unwired: 2 in, 2 out]
  n274 = property on="Rev/Fwd" class="Clust (strict)"("Visible"=w27) -> ()  [unwired: 2 in, 2 out]
  n275 = property on="Camera Settings" class="Clust (strict)"("Visible"=w27) -> ()  [unwired: 2 in, 2 out]
  n276 = local write "DB Camera Config"(w27) -> ()
  n277 = global write "WPI_DashboardLogging Global.vi" "Recording"(w10) -> ()
  n278 = local write "Rec Mode"(w10) -> ()
